vi "To and From Standard Sequence.vi"() -> ()   [LabVIEW 2015, in "Sequence Tests.lvlib"]
uses:
  Sequence Tests.lvlib
  Config/Sequence Config.lvclass
  testing/Sequencer Module tests.lvlib
panel:
  out "error out":errorcluster
  out "Pass":bool
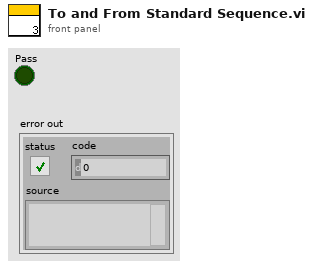
[diagram p1: front panel]
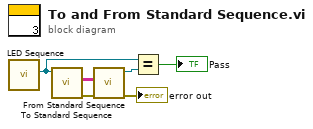
[diagram p0: block diagram]
diagram:
  n1 = call "LED Sequence.vi"() -> ("Sequence out"=w4:refnum<class "Sequence Config.lvclass">)  [unwired: 11 in]
  n2 = call-dynamic "To Standard Sequence.vi"("Sequence Config in"=w4) -> ("error out"=w5:errorcluster, "Standard Sequence"=w6:string[][])  [unwired: 8 in, 1 out]
  n3 = call "From Standard Sequence.vi"("error in (no error)"=w5, "Standard Sequence"=w6) -> ("error out"=→"error out":errorcluster, "Sequence Config.lvclass"=w3:refnum<class "Sequence Config.lvclass">)  [unwired: 8 in]
  n4 = Equal?(x=w4, y=w3) -> (x = y?=→"Pass":bool)
